vi "Benchmarking Time Delay HR.vi"() -> ()   [LabVIEW 2014]
panel:
  in  "stop":bool
  out "Actual Delay (ms)":dbl
  out "Count":i32
  in  "N":i32
  # "Benchmarking Time Delay"
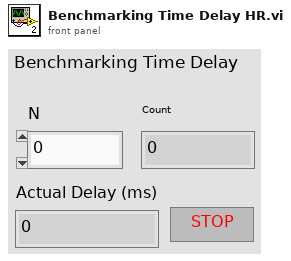
[diagram p1: front panel]
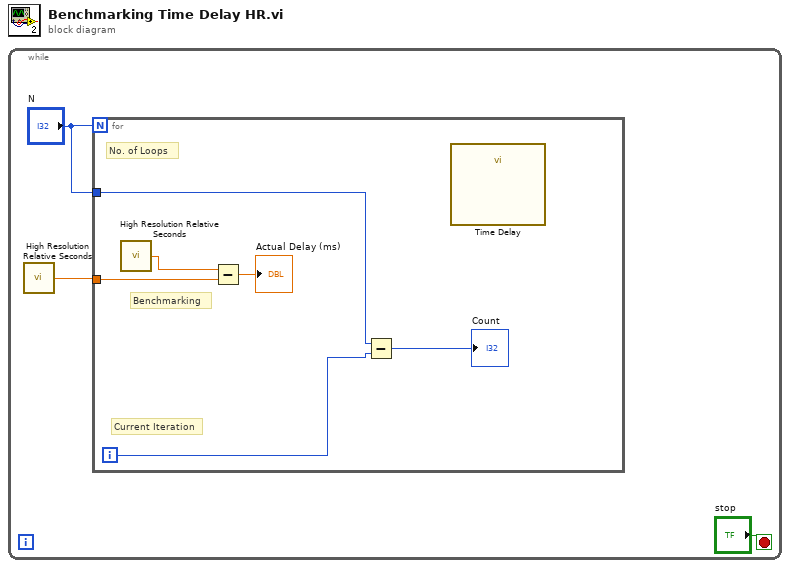
[diagram p0: block diagram]
diagram:
  n1 = while {
    stop <- "stop" stop-if-true
    n2 = call <vilib>:"High Resolution Relative Seconds.vi"() -> ("relative seconds"=w1:dbl)
    n3 = for {
      N: "N" -> [_]
      tunnel: w1 -> [w8]
      tunnel: "N" -> [w7]
      i -> [w5]
      # "Benchmarking"
      # "Current Iteration"
      # "No. of Loops"
      n4 = call <vilib>:"High Resolution Relative Seconds.vi"() -> ("relative seconds"=w4:dbl)
      n5 = Subtract(x=w4, y=w8) -> (x-y=→"Actual Delay (ms)":dbl)
      n6 = Subtract(x=w7, y=w5) -> (x-y=→"Count":i32)
      n7 = call "Time Delay"() -> ()  [unwired: 11 in, 1 out]
    }
  }
